vi "Run Script.vi"(8 "error in (no error)":errorcluster, 10 "Script Name (\"\")":string, 11 "VISA resource name":refnum<visa-resource-name>) -> (0 "error out":errorcluster, 3 "VISA resource name out":refnum<visa-resource-name>)   [LabVIEW 2023, in "Keithley DMM6500 DAQ6500 Series.lvlib"]
doc: "Runs a script."
uses:
  <instrlib>/Keithley DMM6500 DAQ6500 Series/Keithley DMM6500 DAQ6500 Series.lvlib
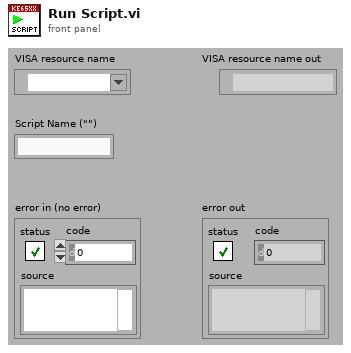
[diagram p1: front panel]
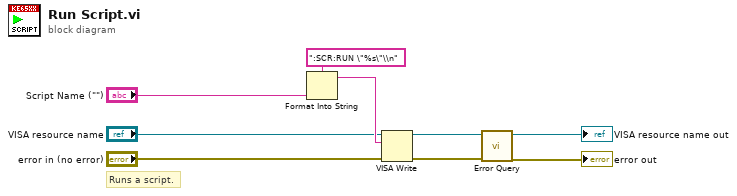
[diagram p0: block diagram]
diagram:
  # "Runs a script."
  n1 = Format Into String(format string=":SCR:RUN \"%s\"\\n", "Script Name (\"\")") -> (resulting string=w7:string)  [unwired: 2 in, 1 out]
  n2 = VISA Write(VISA resource name="VISA resource name", write buffer=w7, error in (no error)="error in (no error)") -> (VISA resource name out=w4:refnum<visa-resource-name>, error out=w3:errorcluster)  [unwired: 1 out]
  n3 = call <instrlib>:"Error Query.vi"("error in (no error)"=w3, "VISA resource name"=w4) -> ("error out"=→"error out":errorcluster, "VISA resource name out"=→"VISA resource name out":refnum<visa-resource-name>)  [unwired: 6 in, 2 out]
